vi "STAT 2 Tractor Decode Digital Data.vi"(0 "Received(T)":bool=TRUE, 7 "Controller SATT 2":T2 {"Tension Sub 2"."sys register" format="%04x"; "Tension Sub 1"."sys register" format="%04x"; "PSU"."sys register" format="%04x"; "solonoid"."valve status" format="%02x"; "solonoid"."sys register" format="%04x"; "pressure 2"."sys register" format="%04x"; "pressure 1"."sys register" format="%04x"; "Controller local"."High G monitoring" format="%02x"; "Controller local"."NA" format="%02x"; "Controller local"."GPIO values" format="%02x"; "Controller local"."Relay status" format="%02x"; "Controller local"."sys register" format="%04x"}, 11 "error in (no error)":errorcluster) -> (6 "Tool digital value":T1[](array[typedef]), 10 "Tool digital indexes":u16[](array[numeric]), 15 "error out":errorcluster)   [LabVIEW 2011]
uses:
  Stroker/Stat def/Stroker system stat2.ctl
  LEINmaster/Nodes/Controller local stat2.ctl
  LEINmaster/Nodes/pressure stat2.ctl
  LEINmaster/Nodes/solonoid stat2.ctl
  LEINmaster/Nodes/PSU stat2.ctl
  LEINmaster/Nodes/tensionsub stat2.ctl
  Measurments Handling/Status Digitalish.ctl
  High Level/Variable List Tractor Digital.ctl
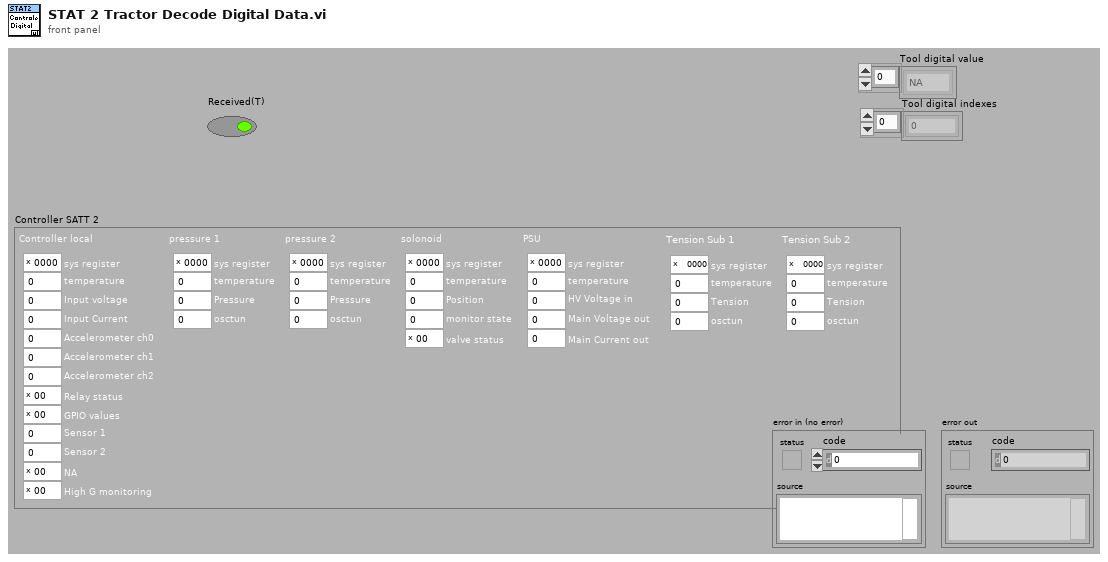
[diagram p1: front panel]
types:
  T1 = typedef "Status Digitalish.ctl" = enum16{"NA", "False", "True"}
  T2 = typedef "Stroker system stat2.ctl" = cluster{"Controller local":T3, "pressure 1":T4, "pressure 2":T4, "solonoid":T5, "PSU":T6, "Tension Sub 1":T7, "Tension Sub 2":T7}
  T3 = typedef "Controller local stat2.ctl" = cluster{"sys register":u16, "temperature":u16, "Input voltage":u16, "Input Current":u16, "Accelerometer ch0":u16, "Accelerometer ch1":u16, "Accelerometer ch2":u16, "Relay status":u8, "GPIO values":u8, "Sensor 1":i32, "Sensor 2":i32, "NA":u8, "High G monitoring":u8}
  T4 = typedef "pressure stat2.ctl" = cluster{"sys register":u16, "temperature":u16, "Pressure":u16, "osctun":u8}
  T5 = typedef "solonoid stat2.ctl" = cluster{"sys register":u16, "temperature":u16, "Position":i16, "monitor state":u8, "valve status":u8}
  T6 = typedef "PSU stat2.ctl" = cluster{"sys register":u16, "temperature":u16, "HV Voltage in":u16, "Main Voltage out":u16, "Main Current out":u16}
  T7 = typedef "tensionsub stat2.ctl" = cluster{"sys register":u16, "temperature":u16, "Tension":i16, "osctun":u8}
  T8 = typedef "Variable List Tractor Digital.ctl" = enum16{"Tractor Relay 1", "Tractor Relay 2", "Tractor Upper Tension Sub", "Tractor Lower Tension Sub", "Tractor Controller error", "Tractor Upper Tension Sub error", "Tractor Lower Tension Sub error", "Tractor Controller stopped", "Tractor Upper Tension Sub stopped", "Tractor Lower Tension Sub stopped"}
  T9 = typedef "Options  All pages and custom.ctl" = cluster{"P 1 (App)":T10, "P 2":T11, "P 3":T12, "P 4":T14, "P 5":T18, "P 6 (Err)":T19, "P 7 (Expert)":T20, "C 1":T22, "C 2":T23}
  T10 = typedef "Options Page 1 (App).ctl" = cluster{"Result files":path, "PCP Interface":string, "Stroker Interface":string, "Tractor Interface":string, "Audible Alarm":bool, "Force alarm on Technical":bool, "Force alarm on HH":bool, "Force alarm on LL":bool, "Force alarm on H":bool, "Force alarm on L":bool}
  T11 = typedef "Options Page 2.ctl" = cluster{"Solenoid & Relay latching time":u16, "Tractor relay 1":dbl, "Tractor relay 2":dbl, "Tractor Solenoid limit":dbl}
  T12 = typedef "Options Page 3.ctl" = cluster{"Min resistance":dbl, "Max resistance":dbl, "PCP/PSU range":T13, "Max voltage jump":dbl, "Maximum resistance change":dbl, "Start Telemetry Voltage":dbl, "Start Telemetry Timeout":dbl, "Start Motor Voltage":dbl, "Stop Motor Voltage":dbl, "Pass Mode Warning Voltage":dbl, "Samples to average":i32}
  T13 = typedef "PCP type List.ctl" = enum16{"0 - 350V", "0 - 450V", "0 - 600V"}
  T14 = typedef "Options Page 4.ctl" = cluster{"Solenoid & Relay latching time":u16, "Stroker relay 1":dbl, "Stroker Relay 2":dbl, "Stroker Solenoid limit":dbl, "Force det.":T15, "Stroke force lim.":dbl, "Pressure SLIPS":dbl, "Tacometer puls":dbl, "Relay Voltage Limit":dbl, "Default anchor behavior":T16, "Default stroker behavior":T17, "Default stroker force limit (tonne)":dbl}
  T15 = typedef "Stroke force selector.ctl" = enum16{"Stroke in = node 1", "Strok out = node 1"}
  T16 = typedef "Default anchor behavior.ctl" = enum16{"Do nothing", "Set Anchor", "Release Anchor"}
  T17 = typedef "Default stroker behavior.ctl" = enum16{"Do nothing", "Stop", "Go Out", "Go In"}
  T18 = typedef "Options Page 5.ctl" = cluster{"Solenoid & Relay latching time":u16, "Driller relay 1":dbl, "Driller Relay 2":dbl, "Driller  Solenoid limit":dbl}
  T19 = typedef "Options Page 6 (Err).ctl" = cluster{"Error and event files":path}
  T20 = typedef "Options Page 7 (Expert).ctl" = cluster{"Show Debug":bool, "Log debug messages":bool, "Aditional debug messages":bool, "enumCANCOM":bool, "AutoLogOn":bool, "Buffer size":i32, "Modem sim":T21, "Modem baud":u16, "Upd regular data":bool, "Show Simulator":bool}
  T21 = typedef "Modem simulation setup.ctl" = cluster{"Modem dealay sim":bool, "Sim baud Tx":u16, "Bit Error fraction Tx":dbl, "Sim baud Rx":u16, "Bit Error fraction Rx":dbl}
  T22 = typedef "Options Custom 1.ctl" = cluster{"Placeholder":bool}
  T23 = typedef "Options Custom 2.ctl" = cluster{"Placeholder":bool}
  T24 = typedef "Stat2 system error.ctl" = cluster{"Error":bool, "Has had error":bool, "Com. issue":bool}
  T25 = typedef "Stat2 system task info.ctl" = cluster{"Task":bool, "Task error":bool, "Task cnt.":u8, "Job 0":bool, "User":bool}
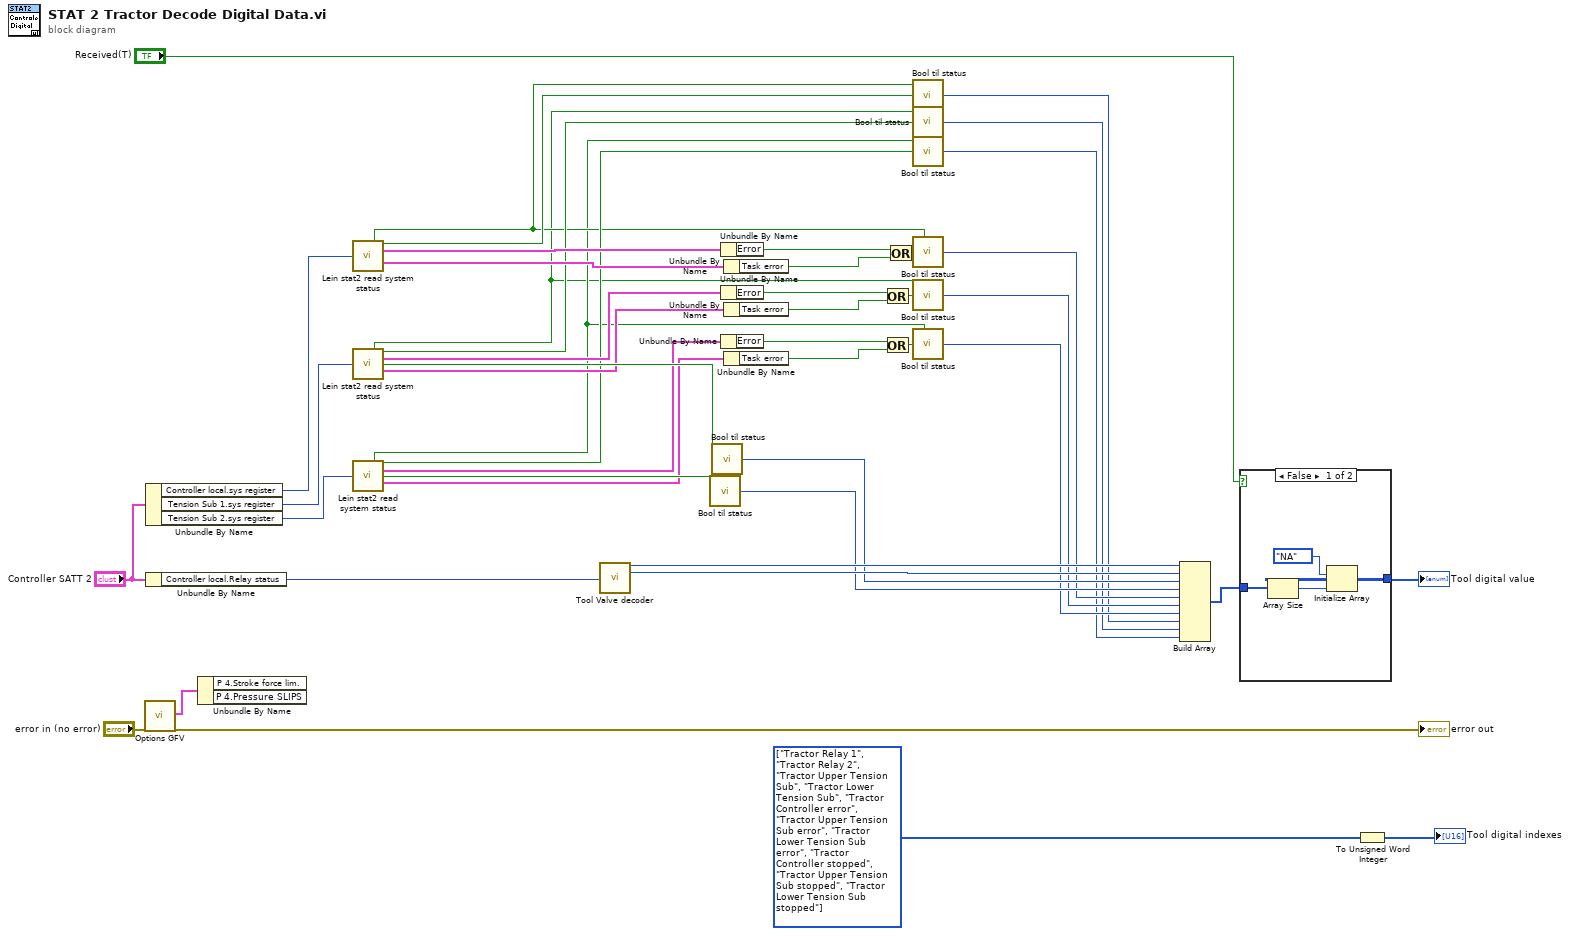
[diagram p0: block diagram]
diagram:
  w1 = T8[] [enum."Tractor Relay 1", enum."Tractor Relay 2", enum."Tractor Upper Tension Sub", enum."Tractor Lower Tension Sub", enum."Tractor Controller error", enum."Tractor Upper Tension Sub error", enum."Tractor Lower Tension Sub error", enum."Tractor Controller stopped", enum."Tractor Upper Tension Sub stopped", enum."Tractor Lower Tension Sub stopped"] items=["Tractor Relay 1", "Tractor Relay 2", "Tractor Upper Tension Sub", "Tractor Lower Tension Sub", "Tractor Controller error", "Tractor Upper Tension Sub error", "Tractor Lower Tension Sub error", "Tractor Controller stopped", "Tractor Upper Tension Sub stopped", "Tractor Lower Tension Sub stopped"]
  n1 = call "Options GFV.vi"("error in (no error)"="error in (no error)") -> ("Options"=w16:T9, "error out"=→"error out":errorcluster)  [unwired: 16 in, 1 out]
  n2 = Unbundle By Name("Controller SATT 2") -> ("Controller local.sys register"=w33:u16, "Tension Sub 1.sys register"=w43:u16, "Tension Sub 2.sys register"=w42:u16)
  n3 = Unbundle By Name("Controller SATT 2") -> ("Controller local.Relay status"=w46:u8)
  n4 = Unbundle By Name(w16) -> ()  [unwired: 2 out]
  n5 = call "Lein stat2 read system status.vi"("sys register"=w33) -> ("Force NA"=w18:bool, "Stopped"=w21:bool, "Error"=w32:T24, "Task"=w30:T25)  [unwired: 7 in, 4 out]
  n6 = call "Lein stat2 read system status.vi"("sys register"=w43) -> ("Force NA"=w12:bool, "Stopped"=w20:bool, "Error"=w37:T24, "Connected"=w40:bool, "Task"=w29:T25)  [unwired: 7 in, 3 out]
  n7 = call "Lein stat2 read system status.vi"("sys register"=w42) -> ("Force NA"=w13:bool, "Stopped"=w19:bool, "Error"=w36:T24, "Connected"=w41:bool, "Task"=w28:T25)  [unwired: 7 in, 3 out]
  n8 = call "Tool Valve decoder.vi"("Valv Relay code"=w46) -> ("Valve LSB(0)"=w45:T1, "Valve 1"=w44:T1)  [unwired: 10 in, 3 out]
  n9 = call "Bool til status.vi"("Boolean"=w41) -> ("Status"=w8:T1)  [unwired: 8 in]
  n10 = call "Bool til status.vi"("Boolean"=w40) -> ("Status"=w9:T1)  [unwired: 8 in]
  n11 = Unbundle By Name(w32) -> ("Error"=w31:bool)
  n12 = Unbundle By Name(w37) -> ("Error"=w35:bool)
  n13 = Unbundle By Name(w36) -> ("Error"=w34:bool)
  n14 = Unbundle By Name(w30) -> ("Task error"=w24:bool)
  n15 = Unbundle By Name(w29) -> ("Task error"=w23:bool)
  n16 = Unbundle By Name(w28) -> ("Task error"=w22:bool)
  n17 = Or(x=w35, y=w23) -> (x .or. y?=w26:bool)
  n18 = Or(x=w34, y=w22) -> (x .or. y?=w27:bool)
  n19 = Or(x=w31, y=w24) -> (x .or. y?=w25:bool)
  n20 = call "Bool til status.vi"("Force NA(F)"=w18, "Boolean"=w21) -> ("Status"=w4:T1)  [unwired: 7 in]
  n21 = call "Bool til status.vi"("Force NA(F)"=w12, "Boolean"=w20) -> ("Status"=w3:T1)  [unwired: 7 in]
  n22 = call "Bool til status.vi"("Force NA(F)"=w13, "Boolean"=w19) -> ("Status"=w2:T1)  [unwired: 7 in]
  n23 = call "Bool til status.vi"("Force NA(F)"=w18, "Boolean"=w25) -> ("Status"=w7:T1)  [unwired: 7 in]
  n24 = call "Bool til status.vi"("Force NA(F)"=w12, "Boolean"=w26) -> ("Status"=w6:T1)  [unwired: 7 in]
  n25 = call "Bool til status.vi"("Force NA(F)"=w13, "Boolean"=w27) -> ("Status"=w5:T1)  [unwired: 7 in]
  n26 = Build Array(w45, w44, w9, w8, w7, w6, w5, w4, w3, w2) -> (w39:T1[])
  n27 = case shown="False" "Received(T)" {
    tunnel: [w48 w51] -> w38
    tunnel: w39 -> [w50 w51]
    frame False {
      n28 = Array Size(array=w50) -> (size(s)=w49:i32)
      n29 = Initialize Array(Status_Digitalish."NA" ("Status"), w49) -> (w48:T1[])
    }
    frame True {
    }
  }
  "Tool digital value" <- w38
  n30 = To Unsigned Word Integer(number=w1) -> (unsigned 16bit integer=→"Tool digital indexes":u16[])
